vi "astrom_test.vi"() -> ()   [LabVIEW 2010]
uses:
  <userlib>/gfitsio/gfitsio.lvlib
panel:
  out "scale (\"/px)":dbl
  out "DEC (°)":dbl
  out "RA (°)":dbl
  in  "Y (px)":dbl
  in  "X (px)":dbl
  in  "Path":path
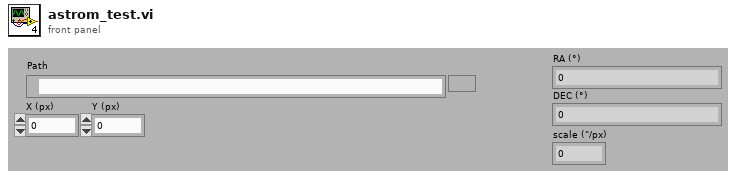
[diagram p1: front panel]
types:
  T1 = typedef "gfitsio.lvlib/gfitsio-refnum.ctl" = refnum<k1>
  T2 = cluster{"NAXIS":dbl[], "CD":dbl[][], "CDELT":dbl[], "CRPIX":dbl[], "CTYPE":string[], "CRVAL":dbl[], "LONGPOLE":dbl, "LATPOLE":dbl, "PV2":dbl[]}
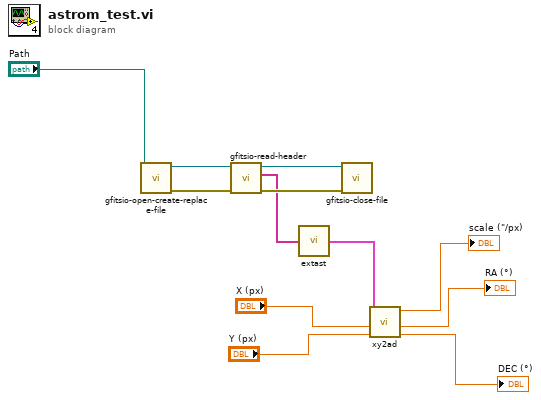
[diagram p0: block diagram]
diagram:
  n1 = call "gfitsio-open-create-replace-file.vi"("file path (dialog if empty)"="Path") -> ("error out"=w10:errorcluster, "gfits refnum"=w11:T1)  [unwired: 8 in, 1 out]
  n2 = call "gfitsio-read-header.vi"("error in (no error)"=w10, "gfits refnum"=w11) -> ("error out"=w8:errorcluster, "header"=w7:string[], "dup gfits refnum"=w9:T1)  [unwired: 7 in]
  n3 = call "extast.vi"("header"=w7) -> ("Astrometry"=w6:T2)  [unwired: 14 in]
  n4 = call <userlib>:"gfitsio-close-file.vi"("error in (no error)"=w8, "gfits refnum"=w9) -> ()  [unwired: 8 in, 2 out]
  n5 = call "xy2ad.vi"("Y (px)"="Y (px)", "X (px)"="X (px)", "Astrometry"=w6) -> ("DEC (°)"=→"DEC (°)":dbl, "RA (°)"=→"RA (°)":dbl, "scale (\"/px)"=→"scale (\"/px)":dbl)  [unwired: 6 in]
